vi "GT Get Event Task Link.vi"(7 "pTaskIndex":i16, 8 "error in (no error)":errorcluster caption="错误输入（无错误）", 9 "pEventIndex":i16, 10 "linkIndex":i16, 11 "cardNum":i16) -> (0 "error out":errorcluster caption="错误输出", 1 "pEventIndex out":i16, 3 "function return":i16, 5 "pTaskIndex out":i16)   [LabVIEW 2020, in "gts1.lvlib"]
doc: "GT_API GT_GetEventTaskLink(short cardNum,short linkIndex,short *pEventIndex,short *pTaskIndex);"
uses:
  gts1.lvlib
  dll/32bit/multi_card/gts.dll
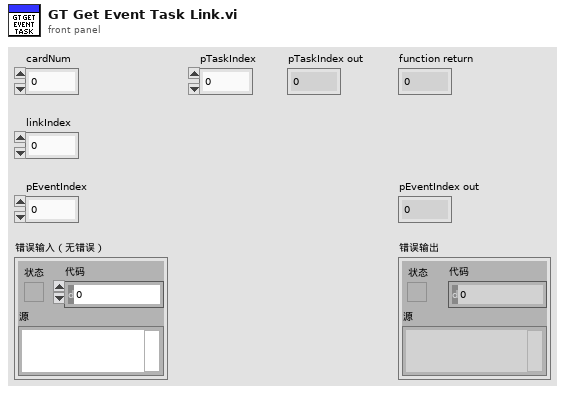
[diagram p1: front panel]
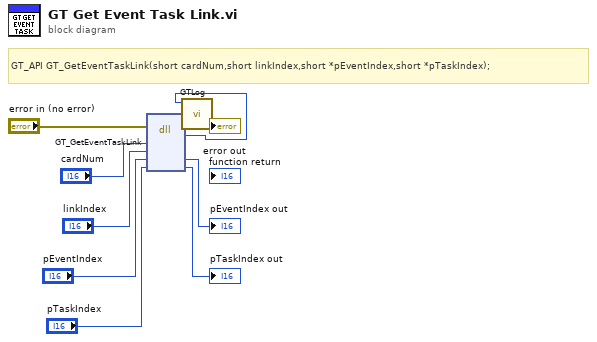
[diagram p0: block diagram]
diagram:
  # "GT_API GT_GetEventTaskLink(short cardNum,short linkIndex,short *pEventIndex,short *pTaskIndex);"
  n1 = dll-call lib="C:/1228/dll/32bit/multi_card/gts.dll" fn="GT_GetEventTaskLink"(error in="error in (no error)", "cardNum"="cardNum", "linkIndex"="linkIndex", "pEventIndex"="pEventIndex", "pTaskIndex"="pTaskIndex") -> (error out=w3:errorcluster, w1:i16, "pEventIndex"=→"pEventIndex out":i16, "pTaskIndex"=→"pTaskIndex out":i16)  [unwired: 4 in, 1 out]
  n2 = call "GTLog.vi"("error in (no error)"=w3, "Numeric"=w1) -> ("error out"=→"error out":errorcluster)  [unwired: 9 in]
